vi "InitPW3390.vi"(4 "DriverOut":refnum<vi>, 6 "DriverIn":refnum<vi>, 8 "error in (no error)":errorcluster, 9 "FetchData":T1, 10 "Power Meter":T2={"Wiring"=0, "Interface"="", "1P Mode"=1, "1P CurrentLimit"=0.0, "3P Mode"=1, "3P CurrentLimit"=0.0} caption="Power Meter BK" {"3P Mode" items=["RMS", "MEAN", "DC"]; "1P Mode" items=["RMS", "MEAN", "DC"]; "Wiring" items=["1P2W", "1P2W+3P3W3M"]}, 11 "PW3390 in":refnum<class "PW3390.lvclass">) -> (0 "error out":errorcluster, 3 "PW3390 out":refnum<class "PW3390.lvclass">)   [LabVIEW 2024, in "PW3390 Actor.lvlib" / "PW3390.lvclass"]
uses:
  PW3390.lvclass
  PW3390.lvclass/PW3390.ctl
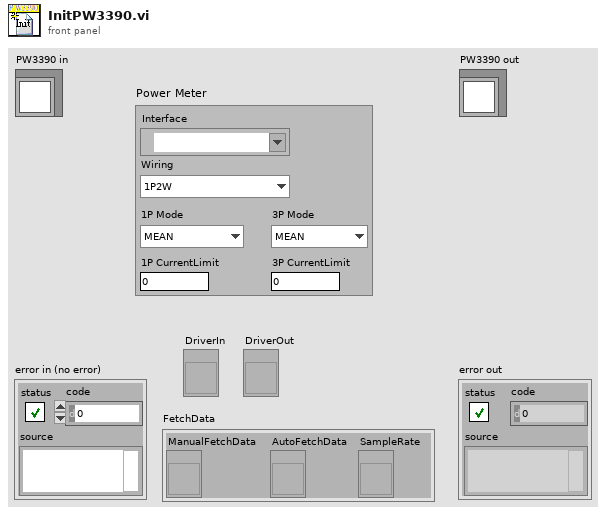
[diagram p1: front panel]
types:
  T1 = cluster{"ManualFetchData":refnum<vi>, "AutoFetchData":refnum<vi>, "SampleRate":refnum<vi>}
  T2 = cluster{"Wiring":u16, "Interface":refnum<visa-resource-name>, "1P Mode":u16, "1P CurrentLimit":dbl, "3P Mode":u16, "3P CurrentLimit":dbl}
  T3 = cluster{"DriverIn":refnum<vi>, "DriverOut":refnum<vi>}
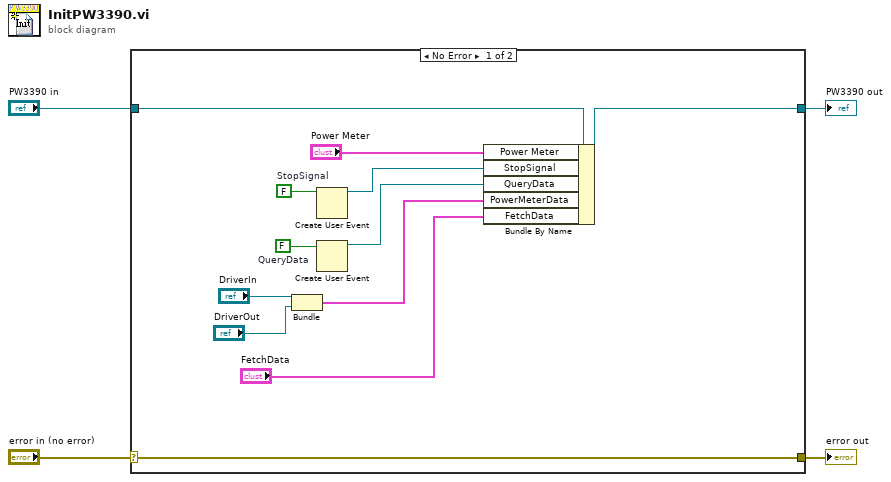
[diagram p0: block diagram]
diagram:
  n1 = case shown="No Error" "error in (no error)" {
    selector: "error in (no error)" -> [w16 w18]
    tunnel: [w16 w18] -> w3
    tunnel: [w10 w17] -> w1
    tunnel: "PW3390 in" -> [w15 w17]
    frame No Error {
      w11 = FALSE  # QueryData
      w13 = FALSE  # StopSignal
      n2 = Bundle("DriverIn"="DriverIn", "DriverOut"="DriverOut") -> (w6:T3)  [unwired: 1 in]
      n3 = Create User Event(user event datatype=w13) -> (user event=w12:refnum<user-event>)  [unwired: 1 in, 1 out]
      n4 = Create User Event(user event datatype=w11) -> (user event=w9:refnum<user-event>)  [unwired: 1 in, 1 out]
      n5 = Bundle By Name(cluster=w15, "Power Meter"="Power Meter", "StopSignal"=w12, "QueryData"=w9, "PowerMeterData"=w6, "FetchData"="FetchData") -> (w10:refnum<class "PW3390.lvclass">)
    }
    frame Error {
    }
  }
  "error out" <- w3
  "PW3390 out" <- w1
